vi "Initialise.vi"(9 "Origin":refnum<class "Vector 2D.lvclass">, 10 "View Size":refnum<class "Vector 2D.lvclass">, 11 "World Size":refnum<class "Vector 2D.lvclass">) -> (3 "Camera out":refnum<class "Camera.lvclass">)   [LabVIEW 2021, in "Camera.lvclass"]
uses:
  Camera.lvclass
  Re-use Libraries/Vector 2D/Vector 2D.lvclass
  Camera.lvclass/Camera.ctl
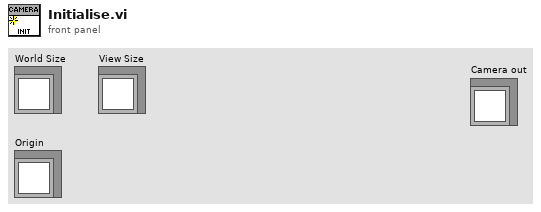
[diagram p1: front panel]
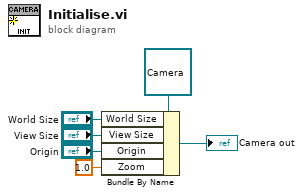
[diagram p0: block diagram]
diagram:
  n1 = Bundle By Name(cluster=refnum<class "Camera.lvclass"> refnum ("Camera in"), "World Size"="World Size", "View Size"="View Size", "Origin"="Origin", "Zoom"=sgl 1.0) -> (→"Camera out":refnum<class "Camera.lvclass">)
